vi "COMMAND DATA.vi"(8 "error in (no error)":errorcluster, 10 "String":string, 11 "action":T1 items=["Initialize Command Store", "Destroy Command Store", "Clear Command  Data", "Append Command  Data", "Get Last Command Data", "Get All Command  Data", "Waiting - Get  Command Data"]) -> (0 "error out":errorcluster, 2 "Command":string, 3 "elements":string[](array[string]))   [LabVIEW 2015, in "Share Variable.lvlib"]
uses:
  Share Variable.lvlib
  COMMAND DATA.ctl
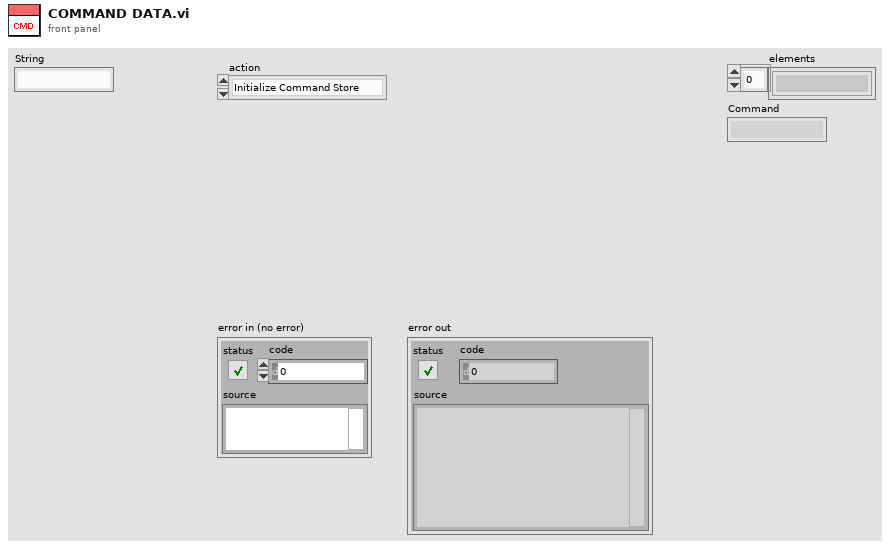
[diagram p1: front panel]
types:
  T1 = typedef "COMMAND DATA.ctl" = u16
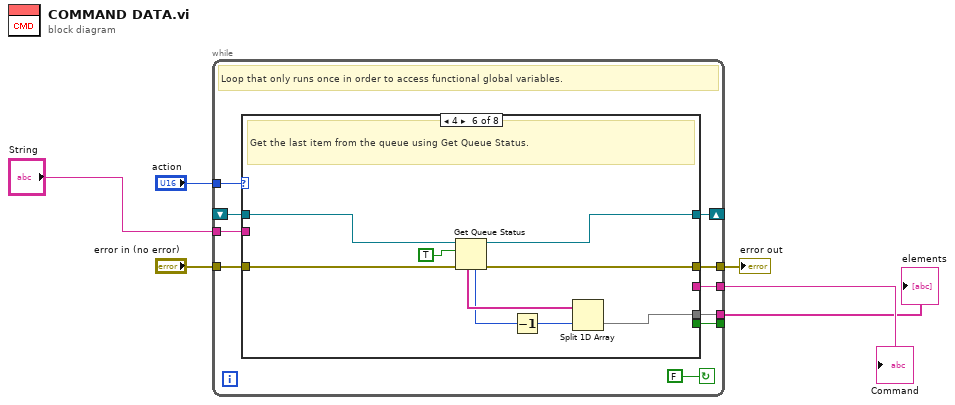
[diagram p0: block diagram]
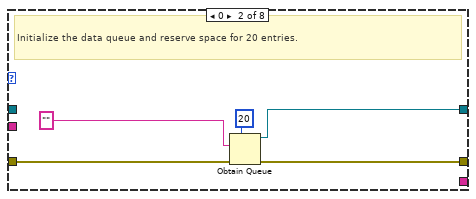
[diagram p3: hidden frame]
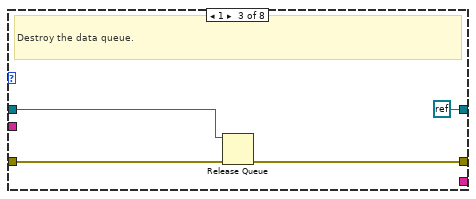
[diagram p4: hidden frame]
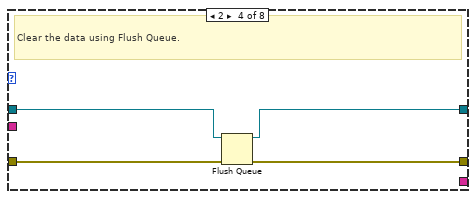
[diagram p5: hidden frame]
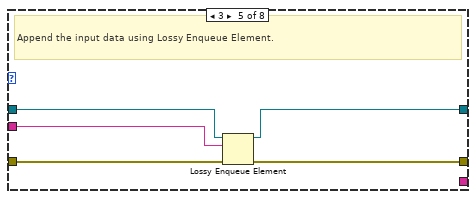
[diagram p6: hidden frame]
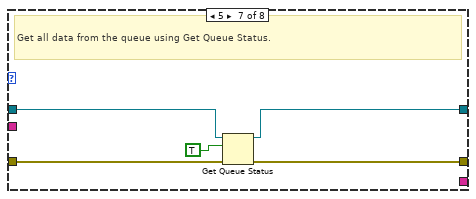
[diagram p7: hidden frame]
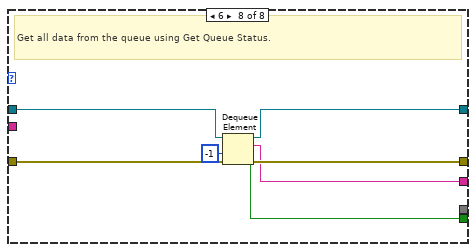
[diagram p8: hidden frame]
diagram:
  n1 = while {
    tunnel: "action" -> [w16]
    shift-right: [w14] -> _
    shift-left: _ -> [w13]
    tunnel: "error in (no error)" -> [w12]
    tunnel: [w11] -> w4
    tunnel: "String" -> [w10]
    tunnel: [w9] -> _
    tunnel: [w8] -> w2
    tunnel: [w7] -> w1
    stop <- FALSE continue-if-true
    # "Loop that only runs once in order to access functional global variables."
    n2 = case shown="4" w16 {
      tunnel: [w18 w23 refnum<k0> refnum w30 w33 w42 w47 w54] -> w14
      tunnel: w13 -> [w18 _ w25 w31 w34 w43 w48 w55]
      tunnel: w12 -> [w17 w21 w27 w29 w36 w45 w50 w57]
      tunnel: [w17 w20 w26 w28 w35 w44 w49 w56] -> w11
      tunnel: w10 -> [_ _ _ _ w32 _ _ _]
      tunnel: [_ _ _ _ _ _ _ w53] -> w9
      tunnel: [_ _ _ _ _ _ _ w51] -> w8
      tunnel: [_ _ _ _ _ w37 _ _] -> w7
      frame Default {
        # "Invalid action."
      }
      frame 0 {
        # "Initialize the data queue and reserve space for 20 entries."
        n3 = Obtain Queue(max queue size (-1, unlimited)=20, element data type="", error in (no error)=w21) -> (queue out=w23:refnum<queue>, error out=w20:errorcluster)  [unwired: 2 in, 1 out]
      }
      frame 1 {
        # "Destroy the data queue."
        n4 = Release Queue(queue=w25, error in (no error)=w27) -> (error out=w26:errorcluster)  [unwired: 1 in, 2 out]
      }
      frame 2 {
        # "Clear the data using Flush Queue."
        n5 = Flush Queue(queue=w31, error in (no error)=w29) -> (queue out=w30:refnum<queue>, error out=w28:errorcluster)  [unwired: 1 out]
      }
      frame 3 {
        # "Append the input data using Lossy Enqueue Element."
        n6 = Lossy Enqueue Element(queue=w34, element=w32, error in (no error)=w36) -> (queue out=w33:refnum<queue>, error out=w35:errorcluster)  [unwired: 2 out]
      }
      frame 4 {
        # "Get the last item from the queue using Get Queue Status."
        n7 = Get Queue Status(queue=w43, return elements? (F)=TRUE, error in (no error)=w45) -> (queue out=w42:refnum<queue>, error out=w44:errorcluster, # elements in queue=w39:i32, elements=w40:string[])  [unwired: 4 out]
        n8 = Decrement(x=w39) -> (x-1=w38:i32)
        n9 = Split 1D Array(array=w40, index=w38) -> (second subarray=w37:string[])  [unwired: 1 out]
      }
      frame 5 {
        # "Get all data from the queue using Get Queue Status."
        n10 = Get Queue Status(queue=w48, return elements? (F)=TRUE, error in (no error)=w50) -> (queue out=w47:refnum<queue>, error out=w49:errorcluster)  [unwired: 6 out]
      }
      frame 6 {
        # "Get all data from the queue using Get Queue Status."
        n11 = Dequeue Element(queue=w55, timeout in ms (-1)=-1, error in (no error)=w57) -> (queue out=w54:refnum<queue>, element=w51:string, timed out?=w53:bool, error out=w56:errorcluster)
      }
    }
  }
  "error out" <- w4
  "elements" <- w1
  "Command" <- w2
